vi "Adjust data window.vi"(6 "dt":dbl, 7 "Channel length":u64, 9 "End, s":dbl=nan format="%.6f", 10 "Start, s":dbl=nan format="%.6f", 11 "Data window":T1={"Start"=0, "Length"=500000, "Channel numbers"=[0], "Channel name"="", "Group name"="Untitled"}) -> ()   [LabVIEW 2015]
uses:
  Data window.ctl
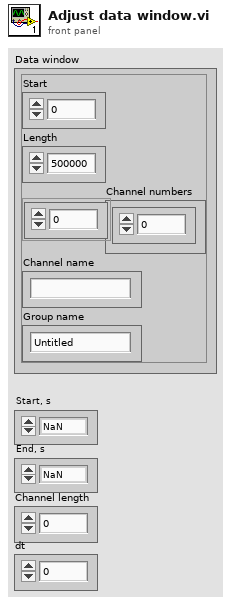
[diagram p1: front panel]
types:
  T1 = typedef "Data window.ctl" = cluster{"Start":i64, "Length":i32, "Channel numbers":i64[], "Channel name":string, "Group name":string}
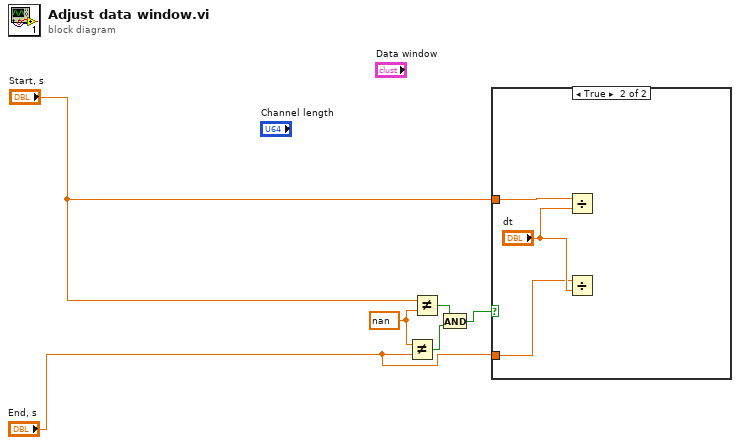
[diagram p0: block diagram]
diagram:
  w6 = nan
  n1 = Not Equal?(x=w6, y="End, s") -> (x != y?=w4:bool)
  n2 = Not Equal?(x="Start, s", y=w6) -> (x != y?=w5:bool)
  n3 = And(x=w5, y=w4) -> (x .and. y?=w3:bool)
  n4 = case shown="True" w3 {
    tunnel: "Start, s" -> [_ w9]
    tunnel: "End, s" -> [_ w7]
    frame False {
    }
    frame True {
      n5 = Divide(x=w9, y="dt") -> ()  [unwired: 1 out]
      n6 = Divide(x=w7, y="dt") -> ()  [unwired: 1 out]
    }
  }
